vi "Update Methods.vi"() -> ()   [LabVIEW 2012]
uses:
  <vilib>/Utility/config.llb/Read Key (Path).vi
  <vilib>/Utility/file.llb/Read From Spreadsheet File (string).vi
  <vilib>/Utility/config.llb/Write Key (Path).vi
  <vilib>/Utility/config.llb/NI_LVConfig.lvlib
panel:
  in  "Modify":bool
  in  "Method Path:":path
  in  "Update":bool
  out "Parameter Table":string[][](table)=[["DG", "50", "50", "50", "50", "50", "50", "100", "100", "50", "50"], ["NG1", "90", "90", "110", "110", "70", "70", "250", "450", "100", "100"], ["HG1", "0", "0", "0", "0", "0", "0", "350", "350", "0", "0"], ["CCP", "0", "400", "0", "400", "0", "420", "420", "420", "0", "430"], ["SX", "500", "500", "500", "500", "500", "500", "500", "500", "500", "500"], ["CD", "0", "0", "0", "0", "0", "0", "0", "2", "0", "0"], ["ISV1", "5850", "5850", "-4400", "-4400", "5850", "5850", "5850", "0", "-4800", "-4800"], ["P1 T", "0", "0", "0", "0", "0", "0", "500", "500", "0", "0"], ["CAP", "1000", "1000", "-1000", "-1000", "1000", "1000", "1000", "1000", "-1000", "-1000"], ["HSID T", "300", "300", "250", "250", "300", "300", "300", "300", "300", "300"], ["EV", "55", "55", "-20", "-20", "30", "30", "30", "30", "-80", "-80"], ["M1 RF", "440", "440", "440", "440", "440", "440", "440", "440", "440", "440"], ["M1", "5", "5", "0", "0", "5", "5", "5", "5", "0", "0"], ["L1", "0", "0", "0", "0", "0", "0", "0", "0", "0", "0"], ["M2", "0", "0", "0", "0", "0", "0", "0", "0", "0", "0"], ["L2", "0", "0", "0", "0", "0", "0", "0", "0", "0", "0"], ["PF", "-15", "-15", "14", "14", "-15", "-15", "-15", "-15", "10", "10"], ["Q1", "-1", "-1", "1", "1", "-1", "-1", "-1", "-1", "1", "1"], ["CCL1", "0", "0", "0", "0", "0", "0", "0", "0", "0", "0"], ["CCL2", "-260", "-60", "320", "50", "-260", "-110", "-110", "-110", "120", "100"], ["CC", "-50", "-20", "130", "12", "-50", "-50", "-50", "-50", "130", "130"], ["CCL3", "-180", "100", "320", "13", "-360", "-51", "-51", "-51", "280", "131"], ["CCL4", "-60", "-60", "50", "35", "-280", "-58.5", "-58.5", "-58.5", "160", "142"], ["CCAF", "100", "100", "-200", "-200", "100", "100", "100", "100", "-200", "-200"], ["Q2", "-100", "-22.5", "132", "14", "-52", "-52", "-52", "-52", "132", "132"], ["ID", "-100", "-140", "90", "120", "-100", "-125", "-125", "-125", "80", "220"], ["DISC", "27", "27", "27", "27", "27", "27", "27", "27", "27", "27"], ["DET horn", "5500", "5500", "5500", "5500", "5500", "5500", "5500", "5500", "5500", "5500"], ["DV", "2000", "2000", "2000", "2000", "2000", "2000", "2000", "2000", "2000", "2000"]]
  in  "Export":bool
  in  "Import":bool
  # "Reserpine Product HF"
  # "T Acid Parent"
  # "Method Name:"
  # "Q1PosPPGs"
  # "Q2PosPPGs"
  # "Q1NegPPGs"
  # "Q2NegPPGs"
  # "Reserpine Parent"
  # "Reserpine Product"
  # "Reserpine Product APCI"
  # "T Acid Product"
  # "1. Modify parameters; 2. Select a method folder; 3. Press update button."
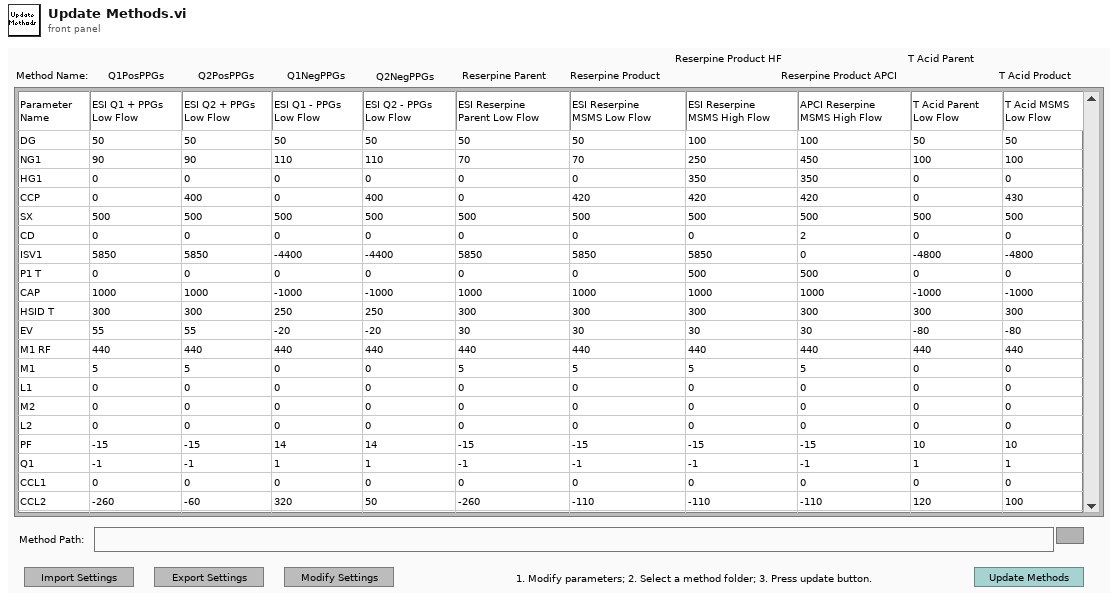
[diagram p1: front panel]
types:
  T1 = enum32{"existing file", "new file", "new or existing file", "existing dir", "new dir", "new or existing dir", "existing file (use LLBs)", "new file (use LLBs)", "new or existing file (use LLBs)", "new or existing file or directory (use LLBs)"}
  T2 = typedef "NI_LVConfig.lvlib/Config Data RefNum.ctl" = refnum<k1>
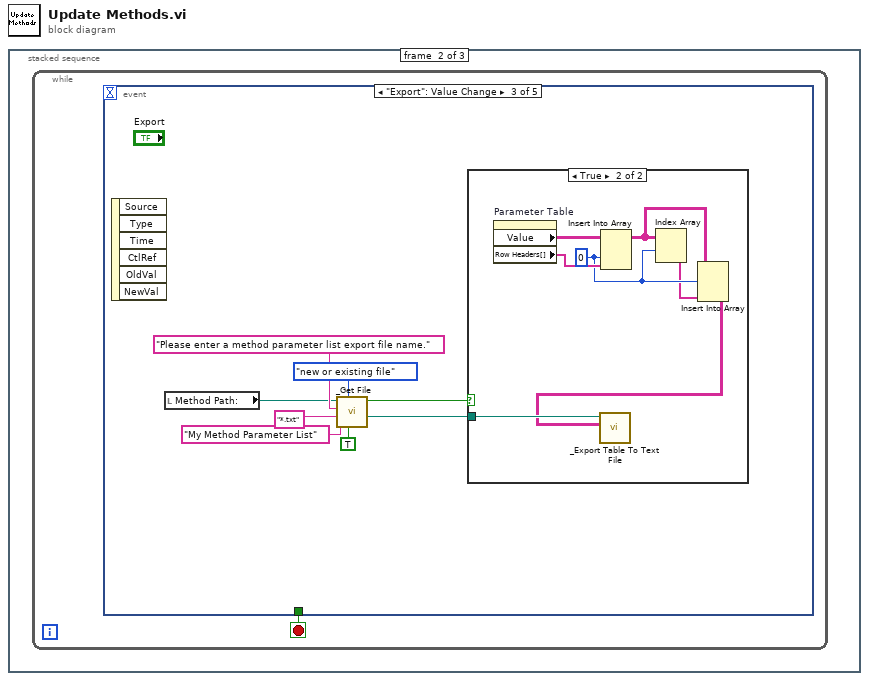
[diagram p0: block diagram]
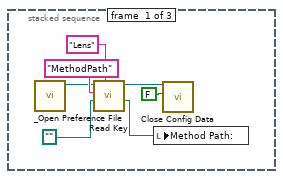
[diagram p2: hidden frame]
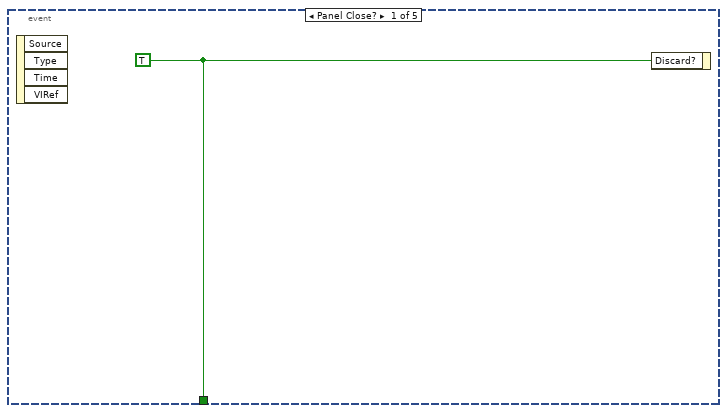
[diagram p3: hidden frame]
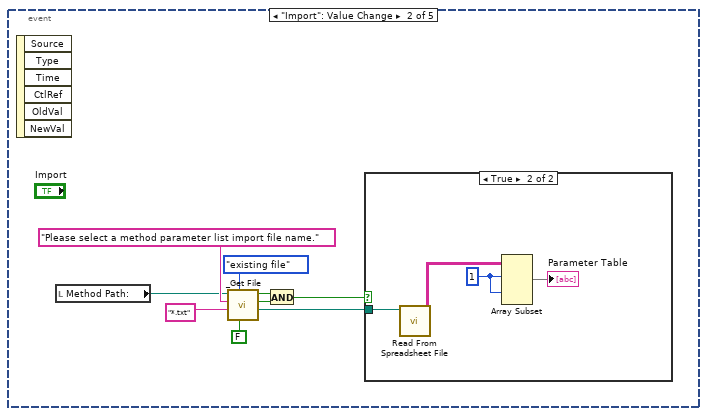
[diagram p4: hidden frame]
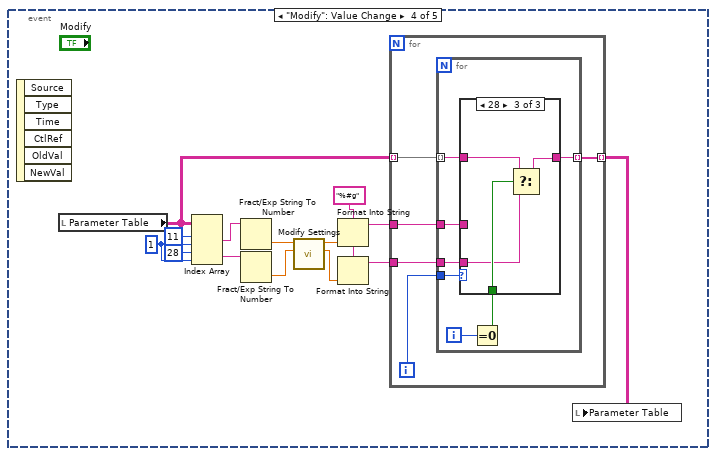
[diagram p7: hidden frame]
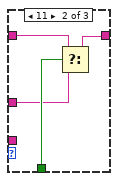
[diagram p9: hidden frame]
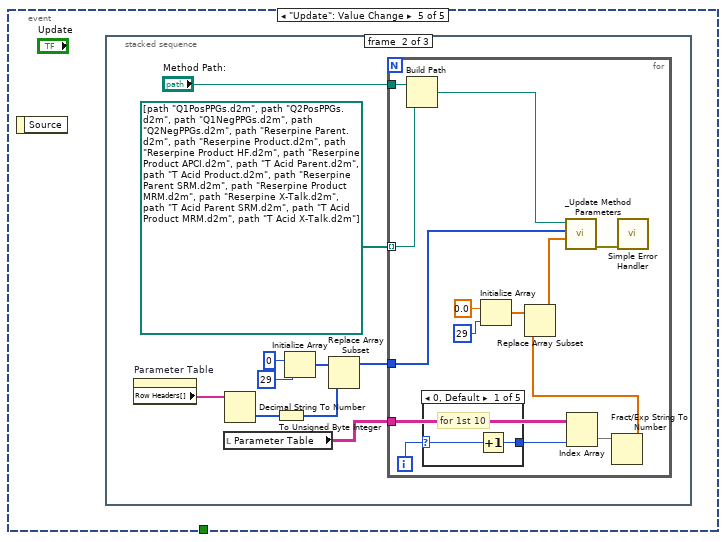
[diagram p10: hidden frame]
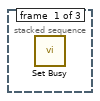
[diagram p11: hidden frame]
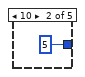
[diagram p12: hidden frame]
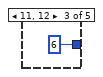
[diagram p13: hidden frame]
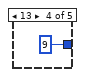
[diagram p14: hidden frame]
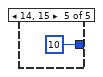
[diagram p15: hidden frame]
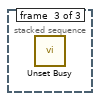
[diagram p16: hidden frame]
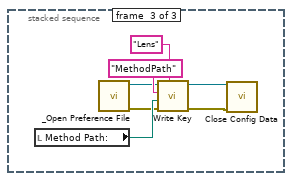
[diagram p17: hidden frame]
diagram:
  n1 = stacked-sequence {
    frame #0 {
      n2 = call "_Open Preference File.vi"() -> ("refnum"=w5:T2)  [unwired: 1 in, 6 out]
      n3 = call-poly <vilib>:"Read Key.vi"("section"="Lens", "default value"=path "", "key"="MethodPath" ("section"), "refnum"=w5) -> ("value"=w1:path, "refnum out"=w3:T2)  [unwired: 1 in, 5 out]
      n4 = local write "Method Path:"(w1) -> ()
      n5 = call <vilib>:"Close Config Data.vi"("write file if changed (T)"=FALSE ("write configuration file? (T)"), "refnum"=w3) -> ()  [unwired: 1 in, 9 out]
    }
    frame #1 {
      n6 = while {
        stop <- w8 stop-if-true
        n7 = event shown="[2] \"Export\": Value Change" {
          selector: _ -> [_ _ _ _ _]
          dyn-events: _ -> [_ _ _ _ _]
          timeout: _ -> [_ _ _ _ _]
          tunnel: [w9 _ _ _ _] -> w8
          event Panel Close? {
            w9 = TRUE ("Discard?")
            n8 = event-data() -> ()  [unwired: 5 out]
            n9 = event-data("Discard?"=w9) -> ()  [unwired: 1 in, 1 out]
          }
          event "Import": Value Change {
            n10 = event-data() -> ()  [unwired: 7 out]
            n11 = local read "Method Path:"() -> (w14:path)
            n12 = call "_Get File.vi"("For Write (T)"=FALSE, "select mode (new or existing)"=T1."existing file", "extension (isd)"="*.txt" ("pattern (all files)"), "prompt"="Please select a method parameter list import file name.", "Start Path"=w14) -> ("Seleted File"=w10:path, "Exists"=w12:bool, "Succeeded"=w13:bool)  [unwired: 1 in, 1 out]
            n13 = And(x=w13, y=w12) -> (x .and. y?=w11:bool)
            n14 = case shown="True" w11 {
              tunnel: w10 -> [_ w22]
              frame False {
              }
              frame True {
                w20 = 1 ("index")
                n15 = call-poly <vilib>:"Read From Spreadsheet File.vi"("file path (dialog if empty)"=w22) -> ("all rows"=w21:string[][])  [unwired: 6 in, 4 out]
                n16 = Array Subset(array=w21, index (row)=w20, index (col)=w20) -> (→"Parameter Table":string[][])  [unwired: 2 in]
              }
            }
          }
          event "Export": Value Change {
            n17 = event-data() -> ()  [unwired: 7 out]
            n18 = local read "Method Path:"() -> (w25:path)
            n19 = call "_Get File.vi"("For Write (T)"=TRUE, "select mode (new or existing)"=T1."new or existing file", "default name"="My Method Parameter List", "extension (isd)"="*.txt" ("pattern (all files)"), "prompt"="Please enter a method parameter list export file name.", "Start Path"=w25) -> ("Seleted File"=w23:path, "Succeeded"=w24:bool)  [unwired: 2 out]
            n20 = case shown="True" w24 {
              tunnel: w23 -> [_ w37]
              frame False {
              }
              frame True {
                w32 = 0 ("index (row)")
                n21 = property on="Parameter Table" class="Tbl (strict)"() -> ("Value"=w35:string[][], "Row Headers[]"=w34:string[])  [unwired: 2 in, 2 out]
                n22 = Insert Into Array(array=w35, index (col)=w32, new element=w34) -> (w33:string[][])  [unwired: 1 in]
                n23 = Index Array(array=w33, index (row)=w32) -> (element=w31:string[])  [unwired: 1 in]
                n24 = Insert Into Array(array=w33, index (row)=w32, new element=w31) -> (w36:string[][])  [unwired: 1 in]
                n25 = call "_Export Table To Text File.vi"("2D data"=w36, "file path (dialog if empty)"=w37) -> ()  [unwired: 4 in, 3 out]
              }
            }
          }
          event "Modify": Value Change {
            w41 = "%#g" ("format string")
            w51 = 1 ("disabled index (col)")
            n26 = event-data() -> ()  [unwired: 7 out]
            n27 = local read "Parameter Table"() -> (w44:string[][])
            n28 = Index Array(array=w44, index (row) #1=11 ("disabled index (row)"), index (col) #1=w51, index (row) #2=28 ("disabled index (row)"), index (col) #2=w51) -> (element #1=w48:string, element #2=w47:string)
            n29 = Fract/Exp String To Number(string=w48) -> (number=w46:dbl)  [unwired: 3 in, 1 out]
            n30 = Fract/Exp String To Number(string=w47) -> (number=w45:dbl)  [unwired: 3 in, 1 out]
            n31 = call "Modify Settings.vi"("DV"=w45, "M1 RF"=w46) -> ("DV 2"=w42:dbl, "M1 RF 2"=w43:dbl)  [unwired: 4 in]
            n32 = Format Into String(format string=w41, w43) -> (resulting string=w39:string)  [unwired: 2 in, 1 out]
            n33 = Format Into String(format string=w41, w42) -> (resulting string=w40:string)  [unwired: 2 in, 1 out]
            n34 = for {
              tunnel: w44 -> [w56] mode=indexing
              tunnel: w40 -> [w54]
              tunnel: w39 -> [w53]
              tunnel: [w52] -> w38 mode=indexing
              i -> [w55]
              n35 = for {
                tunnel: w56 -> [w62] mode=indexing
                tunnel: w55 -> [w63]
                tunnel: w54 -> [w61]
                tunnel: w53 -> [w60]
                tunnel: [w57] -> w52 mode=indexing
                i -> [w59]
                n36 = Equal To 0?(x=w59) -> (x = 0?=w58:bool)
                n37 = case shown="28" w63 {
                  tunnel: [w64 w65 w70] -> w57
                  tunnel: w62 -> [w64 w67 w71]
                  tunnel: w61 -> [_ _ w69]
                  tunnel: w60 -> [_ w66 _]
                  tunnel: w58 -> [_ w68 w72]
                  frame 0, Default {
                  }
                  frame 11 {
                    n38 = Select(t=w67, s=w68, f=w66) -> (s? t:f=w65:string)
                  }
                  frame 28 {
                    n39 = Select(t=w71, s=w72, f=w69) -> (s? t:f=w70:string)
                  }
                }
              }
            }
            n40 = local write "Parameter Table"(w38) -> ()
          }
          event "Update": Value Change {
            n41 = event-data() -> ()  [unwired: 2 out]
            n42 = stacked-sequence {
              frame #0 {
                n43 = call <vilib>:"Set Busy.vi"() -> ()  [unwired: 4 in, 8 out]
              }
              frame #1 {
                n44 = property on="Parameter Table" class="Tbl (strict)"() -> ("Row Headers[]"=w80:string[])  [unwired: 2 in, 2 out]
                n45 = local read "Parameter Table"() -> (w73:string[][])
                n46 = Decimal String To Number(string=w80) -> (number=w79:i32[])  [unwired: 2 in, 1 out]
                n47 = To Unsigned Byte Integer(number=w79) -> (unsigned 8bit integer=w75:u8[])
                n48 = Initialize Array(u8 0 ("element"), 29 ("dimension size")) -> (w77:u8[])
                n49 = Replace Array Subset(array=w77, new element=w75) -> (w74:u8[])  [unwired: 1 in]
                n50 = for {
                  tunnel: path[] [path "Q1PosPPGs.d2m", path "Q2PosPPGs.d2m", path "Q1NegPPGs.d2m", path "Q2NegPPGs.d2m", path "Reserpine Parent.d2m", path "Reserpine Product.d2m", path "Reserpine Product HF.d2m", path "Reserpine Product APCI.d2m", path "T Acid Parent.d2m", path "T Acid Product.d2m", path "Reserpine Parent SRM.d2m", path "Reserpine Product MRM.d2m", path "Reserpine X-Talk.d2m", path "T Acid Parent SRM.d2m", path "T Acid Product MRM.d2m", path "T Acid X-Talk.d2m"] -> [w95] mode=indexing
                  tunnel: "Method Path:" -> [w96]
                  tunnel: w74 -> [w85]
                  tunnel: w73 -> [w84]
                  i -> [w83]
                  n51 = Build Path(base path=w96, name or relative path=w95) -> (appended path=w93:path)
                  n52 = case shown="0, Default" w83 {
                    selector: w83 -> [w97 _ _ _ _]
                    tunnel: [w98 5 6 9 10] -> w94
                    frame 0, Default {
                      # "for 1st 10"
                      n53 = Increment(x=w97) -> (x+1=w98:i32)
                    }
                    frame 10 {
                    }
                    frame 11, 12 {
                    }
                    frame 13 {
                    }
                    frame 14, 15 {
                    }
                  }
                  n54 = Initialize Array(0.0 ("element"), 29 ("dimension size")) -> (w89:dbl[])
                  n55 = Index Array(array=w84, index (col)=w94) -> (element=w92:string[])  [unwired: 1 in]
                  n56 = Fract/Exp String To Number(string=w92) -> (number=w88:dbl[])  [unwired: 3 in, 1 out]
                  n57 = Replace Array Subset(array=w89, new element=w88) -> (w87:dbl[])  [unwired: 1 in]
                  n58 = call "_Update Method Parameters.vi"("Parameter Value"=w87, "Ch#"=w85, "Method File"=w93) -> ("error out"=w91:errorcluster)  [unwired: 8 in]
                  n59 = call <vilib>:"Simple Error Handler.vi"("error in (no error)"=w91) -> ()  [unwired: 4 in, 5 out]
                }
              }
              frame #2 {
                n60 = call <vilib>:"Unset Busy.vi"() -> ()  [unwired: 2 in, 10 out]
              }
            }
          }
        }
      }
    }
    frame #2 {
      n61 = local read "Method Path:"() -> (w105:path)
      n62 = call "_Open Preference File.vi"() -> ("error"=w104:errorcluster, "refnum"=w108:T2)  [unwired: 1 in, 5 out]
      n63 = call-poly <vilib>:"Write Key.vi"("section"="Lens", "error in (no error)"=w104, "value"=w105, "key"="MethodPath" ("section"), "refnum"=w108) -> ("error out"=w103:errorcluster, "refnum out"=w106:T2)  [unwired: 4 in, 1 out]
      n64 = call <vilib>:"Close Config Data.vi"("error in (no error)"=w103, "refnum"=w106) -> ()  [unwired: 1 in, 9 out]
    }
  }
